vi "Pass If.vi"(7 "Description":string, 8 "error in (no error)":errorcluster, 9 "Message":string, 10 "Pass?":bool, 11 "LUnit Test Case In":refnum<class "LUnit Test Case V2.lvclass">) -> (0 "error out":errorcluster, 3 "LUnit Test Case Out":refnum<class "LUnit Test Case V2.lvclass">)   [LabVIEW 2020, in "LUnit Test Case V2.lvclass"]
doc: "Generates a pass result for the calling test method if the conditional input is true. A description and message may be provided."
uses:
  LUnit Test Case V2.lvclass
  Result/Type.ctl
  LUnit Test Case V2.lvclass/LUnit Test Case V2.ctl
  Result/Result.lvlib
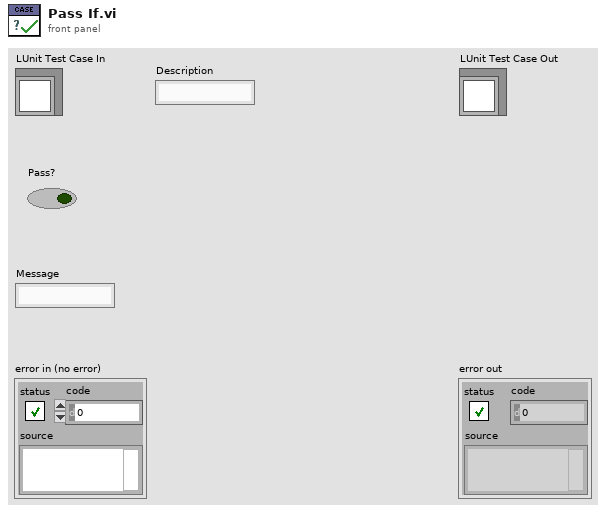
[diagram p1: front panel]
types:
  T1 = typedef "Result.lvlib/Type.ctl" = enum16{"Method", "Case", "Suite", "Pass", "Fail", "Skip", "Pass if", "Fail if", "Pass if Error", "Fail if Error", "Pass if Equal", "Fail if Equal"}
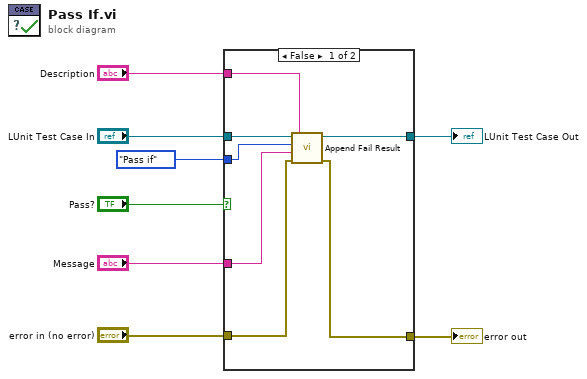
[diagram p0: block diagram]
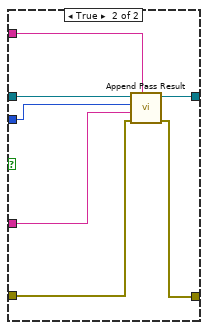
[diagram p2: hidden frame]
diagram:
  n1 = case shown="False" "Pass?" {
    tunnel: [w14 w22] -> w8
    tunnel: [w13 w18] -> w7
    tunnel: "Description" -> [w11 w20]
    tunnel: "Message" -> [w12 w19]
    tunnel: "LUnit Test Case In" -> [w15 w21]
    tunnel: "error in (no error)" -> [w10 w17]
    tunnel: Type."Pass if" ("Result Type") -> [w9 w16]
    frame False {
      n2 = call "Append Fail Result.vi"("Description"=w11, "error in (no error)"=w10, "Message"=w12, "Result Type"=w9, "LUnit Test Case In"=w15) -> ("error out"=w13:errorcluster, "LUnit Test Case Out"=w14:refnum<class "LUnit Test Case V2.lvclass">)  [unwired: 5 in]
    }
    frame True {
      n3 = call "Append Pass Result.vi"("Description"=w20, "error in (no error)"=w17, "Message"=w19, "Result Type"=w16, "LUnit Test Case In"=w21) -> ("error out"=w18:errorcluster, "LUnit Test Case Out"=w22:refnum<class "LUnit Test Case V2.lvclass">)  [unwired: 5 in]
    }
  }
  "error out" <- w7
  "LUnit Test Case Out" <- w8
